vi "ITM10_get_temperature.vi"(7 "channel":i32=1, 8 "err_in":errorcluster, 11 "visa_in":refnum<visa-resource-name>="COM34") -> (0 "err_out":errorcluster={"status"=FALSE, "code"=1073676294, "source"="VISA Read in thcd_get_chan.vi"}, 2 "temp":dbl, 3 "visa_out":refnum<visa-resource-name>="COM3", 4 "status":bool=TRUE, 5 "message":string)   [LabVIEW 2019]
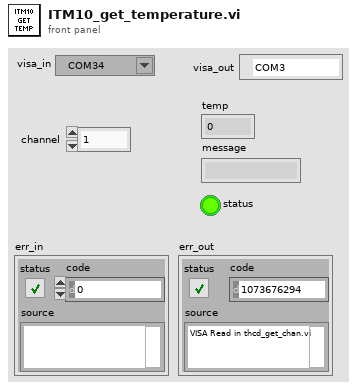
[diagram p1: front panel]
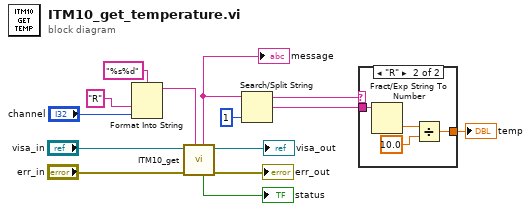
[diagram p0: block diagram]
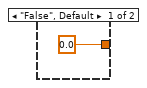
[diagram p2: hidden frame]
diagram:
  n1 = Format Into String(format string="%s%d", "R" ("mks946_comm"), "channel") -> (resulting string=w9:string)  [unwired: 2 in, 1 out]
  n2 = call "ITM10_get.vi"("command"=w9, "error in"="err_in", "VISA_ref_in"="visa_in") -> ("error out"=→"err_out":errorcluster, "VISA_ref_out"=→"visa_out":refnum<visa-resource-name>, "status"=→"status":bool, "response"=w5:string)  [unwired: 5 in]
  "message" <- w5
  n3 = Search/Split String(string=w5, offset (0)=1) -> (substring before match=w3:string, match + rest of string=w2:string)  [unwired: 1 in, 1 out]
  n4 = case shown="\"R\"" w3 {
    tunnel: w2 -> [_ w19]
    tunnel: [0.0 ("value") w18] -> w1
    frame "False", Default {
    }
    frame "R" {
      n5 = Fract/Exp String To Number(string=w19) -> (number=w17:dbl)  [unwired: 3 in, 1 out]
      n6 = Divide(x=w17, y=10.0) -> (x/y=w18:dbl)
    }
  }
  "temp" <- w1
